vi "Power Off Dut.vi"(8 "error in":errorcluster, 11 "Power Sequencing File Path":path) -> (0 "error out":errorcluster)   [LabVIEW 2023]
uses:
  NI gRPC Device Server - Action.ctl
  <instrlib>/niDCPower/nidcpower.llb/niDCPower gRPC Device Server.ctl
  <instrlib>/niDigital/niDigital.llb/niDigital gRPC Device Server.ctl
  <instrlib>/niDigital/niDigital.llb/niDigital Selected Function.ctl
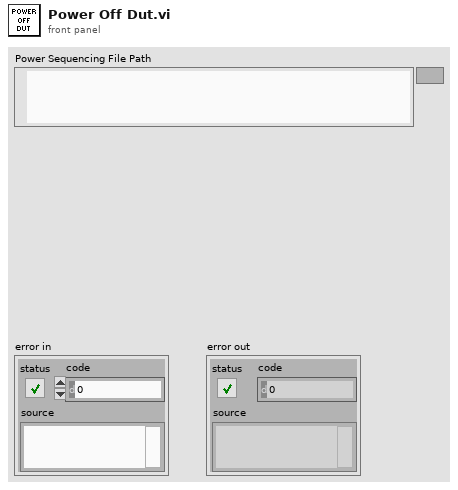
[diagram p1: front panel]
types:
  T1 = typedef "NI gRPC Device Server - Action.ctl" = enum16{"Start Server", "End Server"}
  T2 = typedef "DC Ins Initialize.ctl" = cluster{"Pin Name":string, "Resource Name":refnum<k15>, "Channel":string, "Voltage Range (V)":dbl, "Current Range (A)":dbl, "Instrument Type":T3}
  T3 = typedef "DC Ins Type.ctl" = enum16{"niDigital", "niDCPower", "undefined"}
  T4 = typedef "DC Settings.ctl" = cluster{"Pin Name":string, "Resource Name":refnum<k15>, "Channel":string, "Power-up Seq":u32, "Power-up Voltage (V)":dbl, "Power-down Seq":u32, "Power-down Voltage (V)":dbl, "Current Limit (A)":dbl, "Wait Before Next (ms)":u32, "Instrument Type":T3}
  T5 = typedef "niDCPower gRPC Device Server.ctl" = cluster{"session name":string, "address (localhost)":string, "port (31763)":u32}
  T6 = typedef "niDigital gRPC Device Server.ctl" = cluster{"session name":string, "address (localhost)":string, "port (31763)":u32}
  T7 = typedef "niDigital Selected Function.ctl" = i32
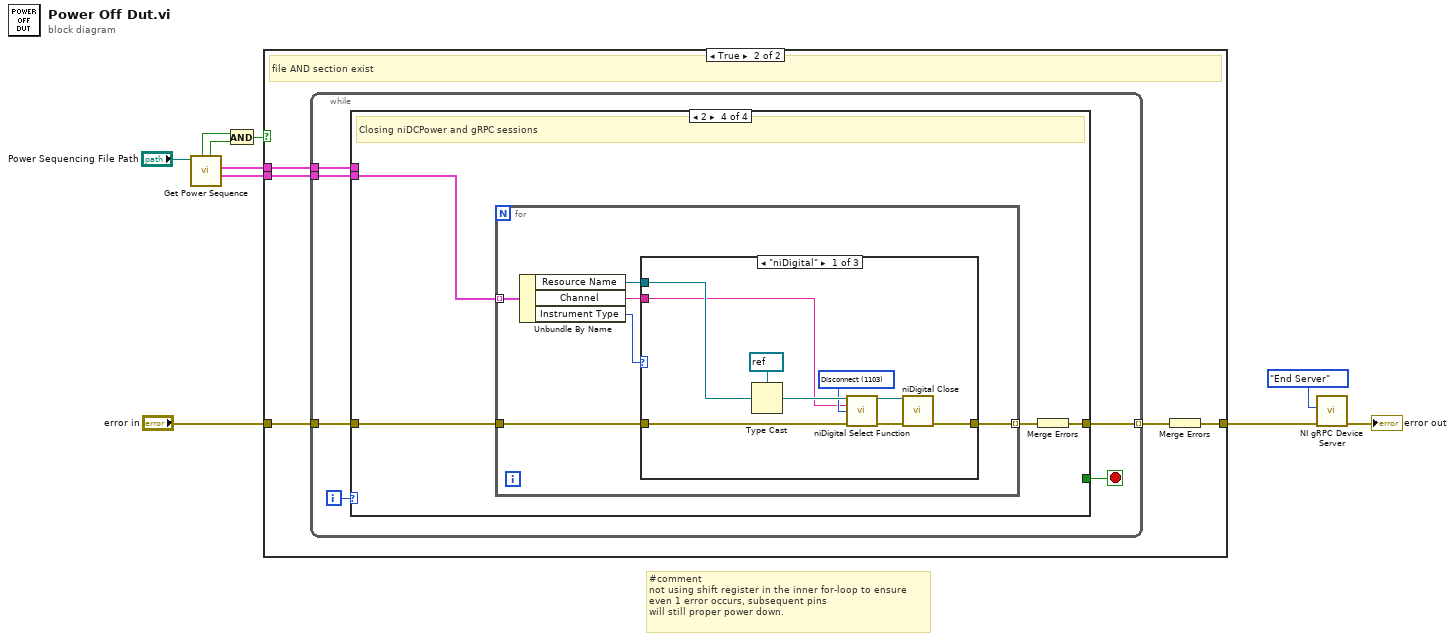
[diagram p0: block diagram]
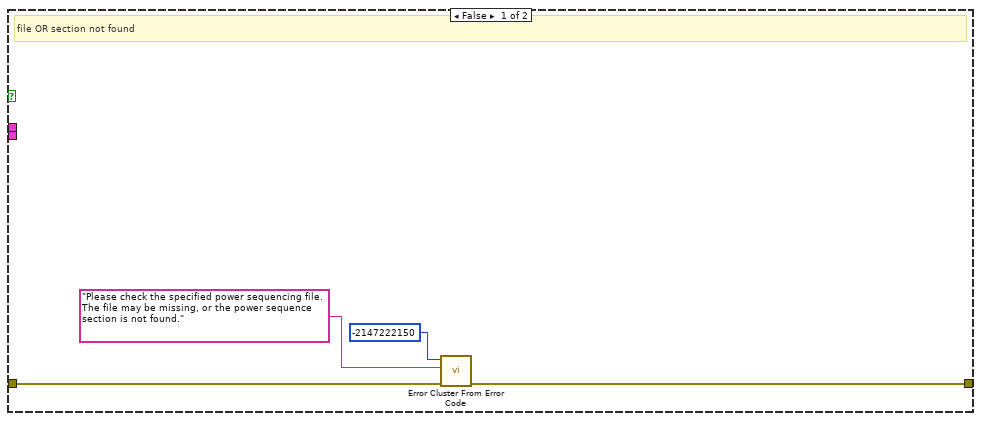
[diagram p2: hidden frame]
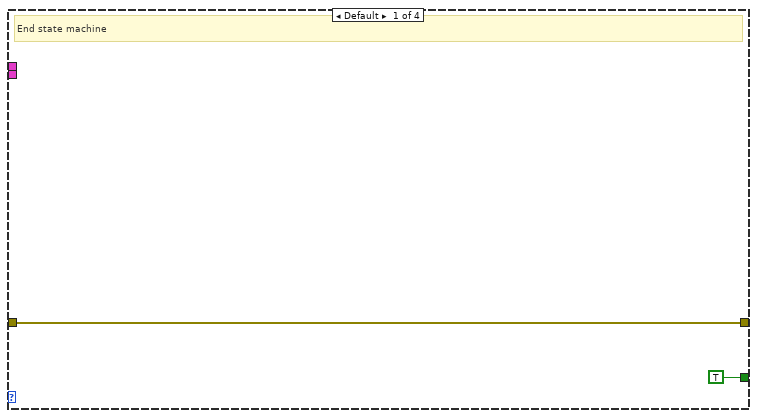
[diagram p3: hidden frame]
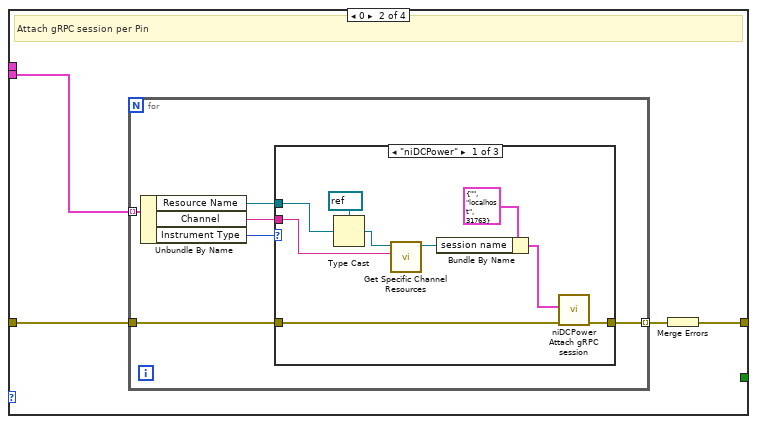
[diagram p4: hidden frame]
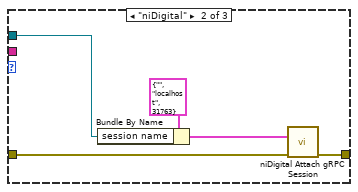
[diagram p5: hidden frame]
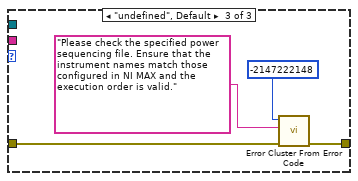
[diagram p6: hidden frame]
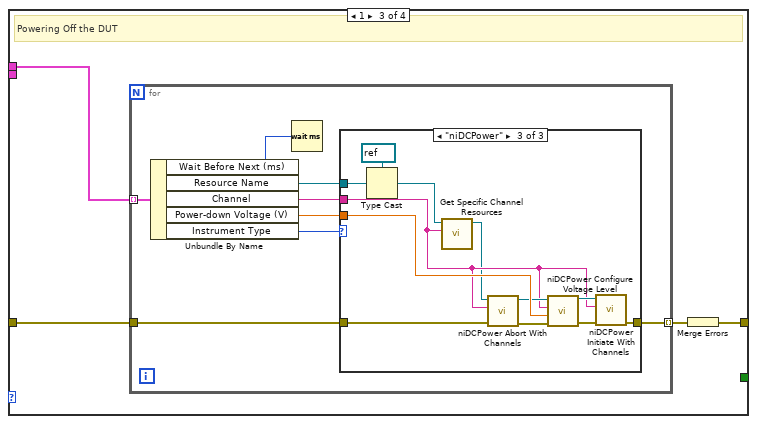
[diagram p7: hidden frame]
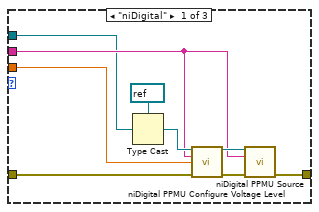
[diagram p8: hidden frame]
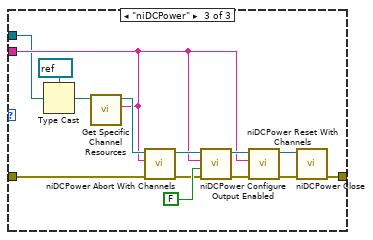
[diagram p11: hidden frame]
diagram:
  # "#comment\nnot using shift register in the inner for-loop to ensure\neven 1 error occurs, subsequent pins\nwill still proper power down."
  n1 = call "Get Power Sequence.vi"("File Path"="Power Sequencing File Path") -> ("SMUs to Initialize (not in order)"=w10:T2[], "Power down Seq"=w9:T4[], "File Exists?"=w7:bool, "Section Exists?"=w6:bool)  [unwired: 6 in, 1 out]
  n2 = And(x=w6, y=w7) -> (x .and. y?=w1:bool)
  n3 = case shown="True" w1 {
    tunnel: w10 -> [_ w18]
    tunnel: w9 -> [_ w17]
    tunnel: "error in" -> [w12 w19]
    tunnel: [w11 w15] -> w4
    frame False {
      # "file OR section not found"
      n4 = call <vilib>:"Error Cluster From Error Code.vi"("error in (no error)"=w12, "error message (\"\")"="Please check the specified power sequencing file. The file may be missing, or the power sequence section is not found.", "error code (0)"=-2147222150) -> ("error out"=w11:errorcluster)  [unwired: 6 in]
    }
    frame True {
      # "file AND section exist"
      n5 = while {
        tunnel: w19 -> [w24]
        tunnel: w18 -> [w22]
        tunnel: w17 -> [w21]
        tunnel: [w20] -> w16 mode=indexing
        i -> [w25]
        stop <- w23 stop-if-true
        n6 = case shown="2" w25 {
          tunnel: w24 -> [w26 w31 w59 w93]
          tunnel: [TRUE _ _ _] -> w23
          tunnel: w22 -> [_ w30 _ w92]
          tunnel: w21 -> [_ _ w58 _]
          tunnel: [w26 w28 w56 w90] -> w20
          frame Default {
            # "End state machine"
          }
          frame 0 {
            # "Attach gRPC session per Pin"
            n7 = for {
              tunnel: w30 -> [w37] mode=indexing
              tunnel: w31 -> [w34]
              tunnel: [w33] -> w29 mode=indexing
              # "Attach gRPC session per Pin"
              n8 = Unbundle By Name(w37) -> ("Resource Name"=w36:refnum<k15>, "Channel"=w35:string, "Instrument Type"=w32:T3)
              n9 = case shown="\"niDCPower\"" w32 {
                tunnel: w36 -> [w38 w47 _]
                tunnel: w35 -> [w46 _ _]
                tunnel: w34 -> [w42 w49 w53]
                tunnel: [w41 w48 w52] -> w33
                frame "niDCPower" {
                  n10 = Type Cast(type=refnum<k15> refnum ("Resource Name"), x=w38) -> (*(type *) &x=w39:refnum<k15>)
                  n11 = call "Get Specific Channel Resources.vi"("Channel"=w46, "Resource Name"=w39) -> ("Resource Name"=w44:refnum<k15>)  [unwired: 9 in]
                  n12 = Bundle By Name(cluster=T5 {"session name"="", "address (localhost)"="localhost", "port (31763)"=31763} ("gRPC options"), "session name"=w44) -> (w43:T5)
                  n13 = call <instrlib>:"niDCPower Attach gRPC session.vi"("error in (no error)"=w42, "gRPC options"=w43) -> ("error out"=w41:errorcluster)  [unwired: 8 in, 1 out]
                }
                frame "niDigital" {
                  n14 = Bundle By Name(cluster=T6 {"session name"="", "address (localhost)"="localhost", "port (31763)"=31763} ("gRPC options"), "session name"=w47) -> (w50:T6)
                  n15 = call <instrlib>:"niDigital Attach gRPC Session.vi"("gRPC options"=w50, "error in"=w49) -> ("error out"=w48:errorcluster)  [unwired: 12 in, 1 out]
                }
                frame "undefined", Default {
                  n16 = call <vilib>:"Error Cluster From Error Code.vi"("error in (no error)"=w53, "error message (\"\")"="Please check the specified power sequencing file. Ensure that the instrument names match those configured in NI MAX and the execution order is valid." ("error message (\"\")"), "error code (0)"=-2147222148) -> ("error out"=w52:errorcluster)  [unwired: 6 in]
                }
              }
            }
            n17 = Merge Errors(w29) -> (w28:errorcluster)
          }
          frame 1 {
            # "Powering Off the DUT"
            n18 = for {
              tunnel: w58 -> [w65] mode=indexing
              tunnel: w59 -> [w61]
              tunnel: [w63] -> w57 mode=indexing
              # "Powering Off the DUT"
              n19 = Unbundle By Name(w65) -> ("Wait Before Next (ms)"=w66:u32, "Resource Name"=w67:refnum<k15>, "Channel"=w62:string, "Power-down Voltage (V)"=w64:dbl, "Instrument Type"=w60:T3)
              n20 = Wait (ms)(milliseconds to wait=w66) -> ()  [unwired: 1 out]
              n21 = case shown="\"niDCPower\"" w60 {
                tunnel: w67 -> [w69 _ w79]
                tunnel: w64 -> [w68 _ w89]
                tunnel: [w71 w77 w85] -> w63
                tunnel: w62 -> [w70 _ w83]
                tunnel: w61 -> [w72 w77 w82]
                frame "niDigital" {
                  n22 = Type Cast(type=refnum<k15> refnum ("instrument handle"), x=w69) -> (*(type *) &x=w74:refnum<k15>)
                  n23 = call <instrlib>:"niDigital PPMU Configure Voltage Level.vi"("instrument handle"=w74, "channel list"=w70, "voltage level (V)"=w68, "error in"=w72) -> ("instrument handle out"=w75:refnum<k15>, "error out"=w76:errorcluster)  [unwired: 10 in]
                  n24 = call <instrlib>:"niDigital PPMU Source.vi"("instrument handle"=w75, "channel list"=w70, "error in"=w76) -> ("error out"=w71:errorcluster)  [unwired: 11 in, 1 out]
                }
                frame "undefined", Default {
                }
                frame "niDCPower" {
                  n25 = Type Cast(type=refnum<k15> refnum ("Resource Name"), x=w79) -> (*(type *) &x=w78:refnum<k15>)
                  n26 = call "Get Specific Channel Resources.vi"("Channel"=w83, "Resource Name"=w78) -> ("Resource Name"=w81:refnum<k15>)  [unwired: 9 in]
                  n27 = call <instrlib>:"niDCPower Abort With Channels.vi"("error in (no error)"=w82, "channel name"=w83, "instrument handle"=w81) -> ("error out"=w88:errorcluster, "instrument handle out"=w87:refnum<k15>)  [unwired: 7 in]
                  n28 = call <instrlib>:"niDCPower Configure Voltage Level.vi"("error in (no error)"=w88, "voltage level"=w89, "channel name"=w83, "instrument handle"=w87) -> ("error out"=w86:errorcluster, "instrument handle out"=w84:refnum<k15>)  [unwired: 6 in]
                  n29 = call <instrlib>:"niDCPower Initiate With Channels.vi"("error in (no error)"=w86, "channel name"=w83, "instrument handle"=w84) -> ("error out"=w85:errorcluster)  [unwired: 7 in, 1 out]
                }
              }
            }
            n30 = Merge Errors(w57) -> (w56:errorcluster)
          }
          frame 2 {
            # "Closing niDCPower and gRPC sessions"
            n31 = for {
              tunnel: w92 -> [w98] mode=indexing
              tunnel: w93 -> [w97]
              tunnel: [w95] -> w91 mode=indexing
              # "Closing niDCPower and gRPC sessions"
              n32 = Unbundle By Name(w98) -> ("Resource Name"=w99:refnum<k15>, "Channel"=w96:string, "Instrument Type"=w94:T3)
              n33 = case shown="\"niDigital\"" w94 {
                tunnel: w99 -> [w101 _ w110]
                tunnel: w97 -> [w102 w109 w119]
                tunnel: w96 -> [w100 _ w114]
                tunnel: [w103 w109 w113] -> w95
                frame "niDigital" {
                  w105 = T7 1103 items=["Digital"=1100, "PPMU"=1101, "Off"=1102, "Disconnect"=1103] ("function")
                  n34 = Type Cast(type=refnum<k15> refnum ("instrument handle"), x=w101) -> (*(type *) &x=w108:refnum<k15>)
                  n35 = call <instrlib>:"niDigital Select Function.vi"("instrument handle"=w108, "channel list"=w100, "function"=w105, "error in"=w102) -> ("instrument handle out"=w106:refnum<k15>, "error out"=w107:errorcluster)  [unwired: 10 in]
                  n36 = call <instrlib>:"niDigital Close.vi"("instrument handle"=w106, "error in"=w107) -> ("error out"=w103:errorcluster)  [unwired: 13 in]
                }
                frame "undefined", Default {
                }
                frame "niDCPower" {
                  n37 = Type Cast(type=refnum<k15> refnum ("Resource Name"), x=w110) -> (*(type *) &x=w111:refnum<k15>)
                  n38 = call "Get Specific Channel Resources.vi"("Channel"=w114, "Resource Name"=w111) -> ("Resource Name"=w120:refnum<k15>)  [unwired: 9 in]
                  n39 = call <instrlib>:"niDCPower Abort With Channels.vi"("error in (no error)"=w119, "channel name"=w114, "instrument handle"=w120) -> ("error out"=w117:errorcluster, "instrument handle out"=w118:refnum<k15>)  [unwired: 7 in]
                  n40 = call <instrlib>:"niDCPower Configure Output Enabled.vi"("error in (no error)"=w117, "output enabled"=FALSE, "channel name"=w114, "instrument handle"=w118) -> ("error out"=w115:errorcluster, "instrument handle out"=w116:refnum<k15>)  [unwired: 6 in]
                  n41 = call <instrlib>:"niDCPower Reset With Channels.vi"("error in (no error)"=w115, "channel name"=w114, "instrument handle"=w116) -> ("error out"=w122:errorcluster, "instrument handle out"=w123:refnum<k15>)  [unwired: 7 in]
                  n42 = call <instrlib>:"niDCPower Close.vi"("error in (no error)"=w122, "instrument handle"=w123) -> ("error out"=w113:errorcluster)  [unwired: 9 in]
                }
              }
            }
            n43 = Merge Errors(w91) -> (w90:errorcluster)
          }
        }
      }
      n44 = Merge Errors(w16) -> (w15:errorcluster)
    }
  }
  n45 = call "NI gRPC Device Server.vi"("error in"=w4, "Action"=NI_gRPC_Device_Server_-_Action."End Server") -> ("error out"=→"error out":errorcluster)  [unwired: 9 in]
